vi "Laser.vi"() -> ()   [LabVIEW 2013]
doc: "Пограмма управления мишенью лазерного источника ионов."
uses:
  <vilib>/Utility/error.llb/DialogType.ctl
  <vilib>/Utility/inputDevices.llb/closeJoystick.vi
  <vilib>/Utility/inputDevices.llb/mouseAcquire.vi
panel:
  in  "?":enum32{" Графики", " Настройки соединения"}(tab)
  in  "LiF 3":picture
  in  "LiF 2":picture
  in  "LiF 1":picture
  in  "Дейтерированный полиэтилен":picture
  out "Slide X axis":u8(slide) max=100 scale=0.0..100.0
  out "Slide Y axis":u8(slide) max=50 step=1
  in  "Add Button":bool
  in  "Коорд. Y":u16
  in  "Коорд. X":u16
  in  "Снимок":bool
  in  "Запись в файл":bool
  out "con err":bool caption="Connect"
  out "Con":bool
  out "warning1":string
  out "TCP read data":string
  in  "thickness":u16 step=1
  out "Mouse on Pane pos Horizontal":i32
  out "Mouse on Pane pos Vertical":i32
  out "bytes written":i32
  in  "порт":u16=10001
  in  "IP-адрес":string="159.93.126.157"
  in  "Disconnect":bool caption="Disconn"
  out "Connected":bool
  in  "Connect":bool
  out "TCP error source":string
  in  "stop":bool
  out "read_error_indicator":bool
  in  "Connect 2":bool caption="Connect"
  in  "Компактный вид":bool
  out "resize Fl":bool caption="Disconn"
  in  "flag1":bool caption="Disconn"
  out "x+1":dbl
  out "TCP con ID":refnum<k5>
  # "Дейтерированный полиэтилен"
  # "LiF 1"
  # "LiF 2"
  # "Графит"
types:
  T1 = typedef "DialogType.ctl" = u16
  T2 = typedef "imagedata.ctl" = cluster{"image type":i32, "image depth":i32, "image":u8[], "mask":u8[], "colors":u32[], "Rectangle":cluster{"left":i16, "top":i16, "right":i16, "bottom":i16}}
  T3 = cluster{"Horizontal":i32, "Vertical":i32, "Scrolling":i32}
  T4 = typedef "LVRectTypeDef.ctl" = cluster{"Left":i16, "Top":i16, "Right":i16, "Bottom":i16}
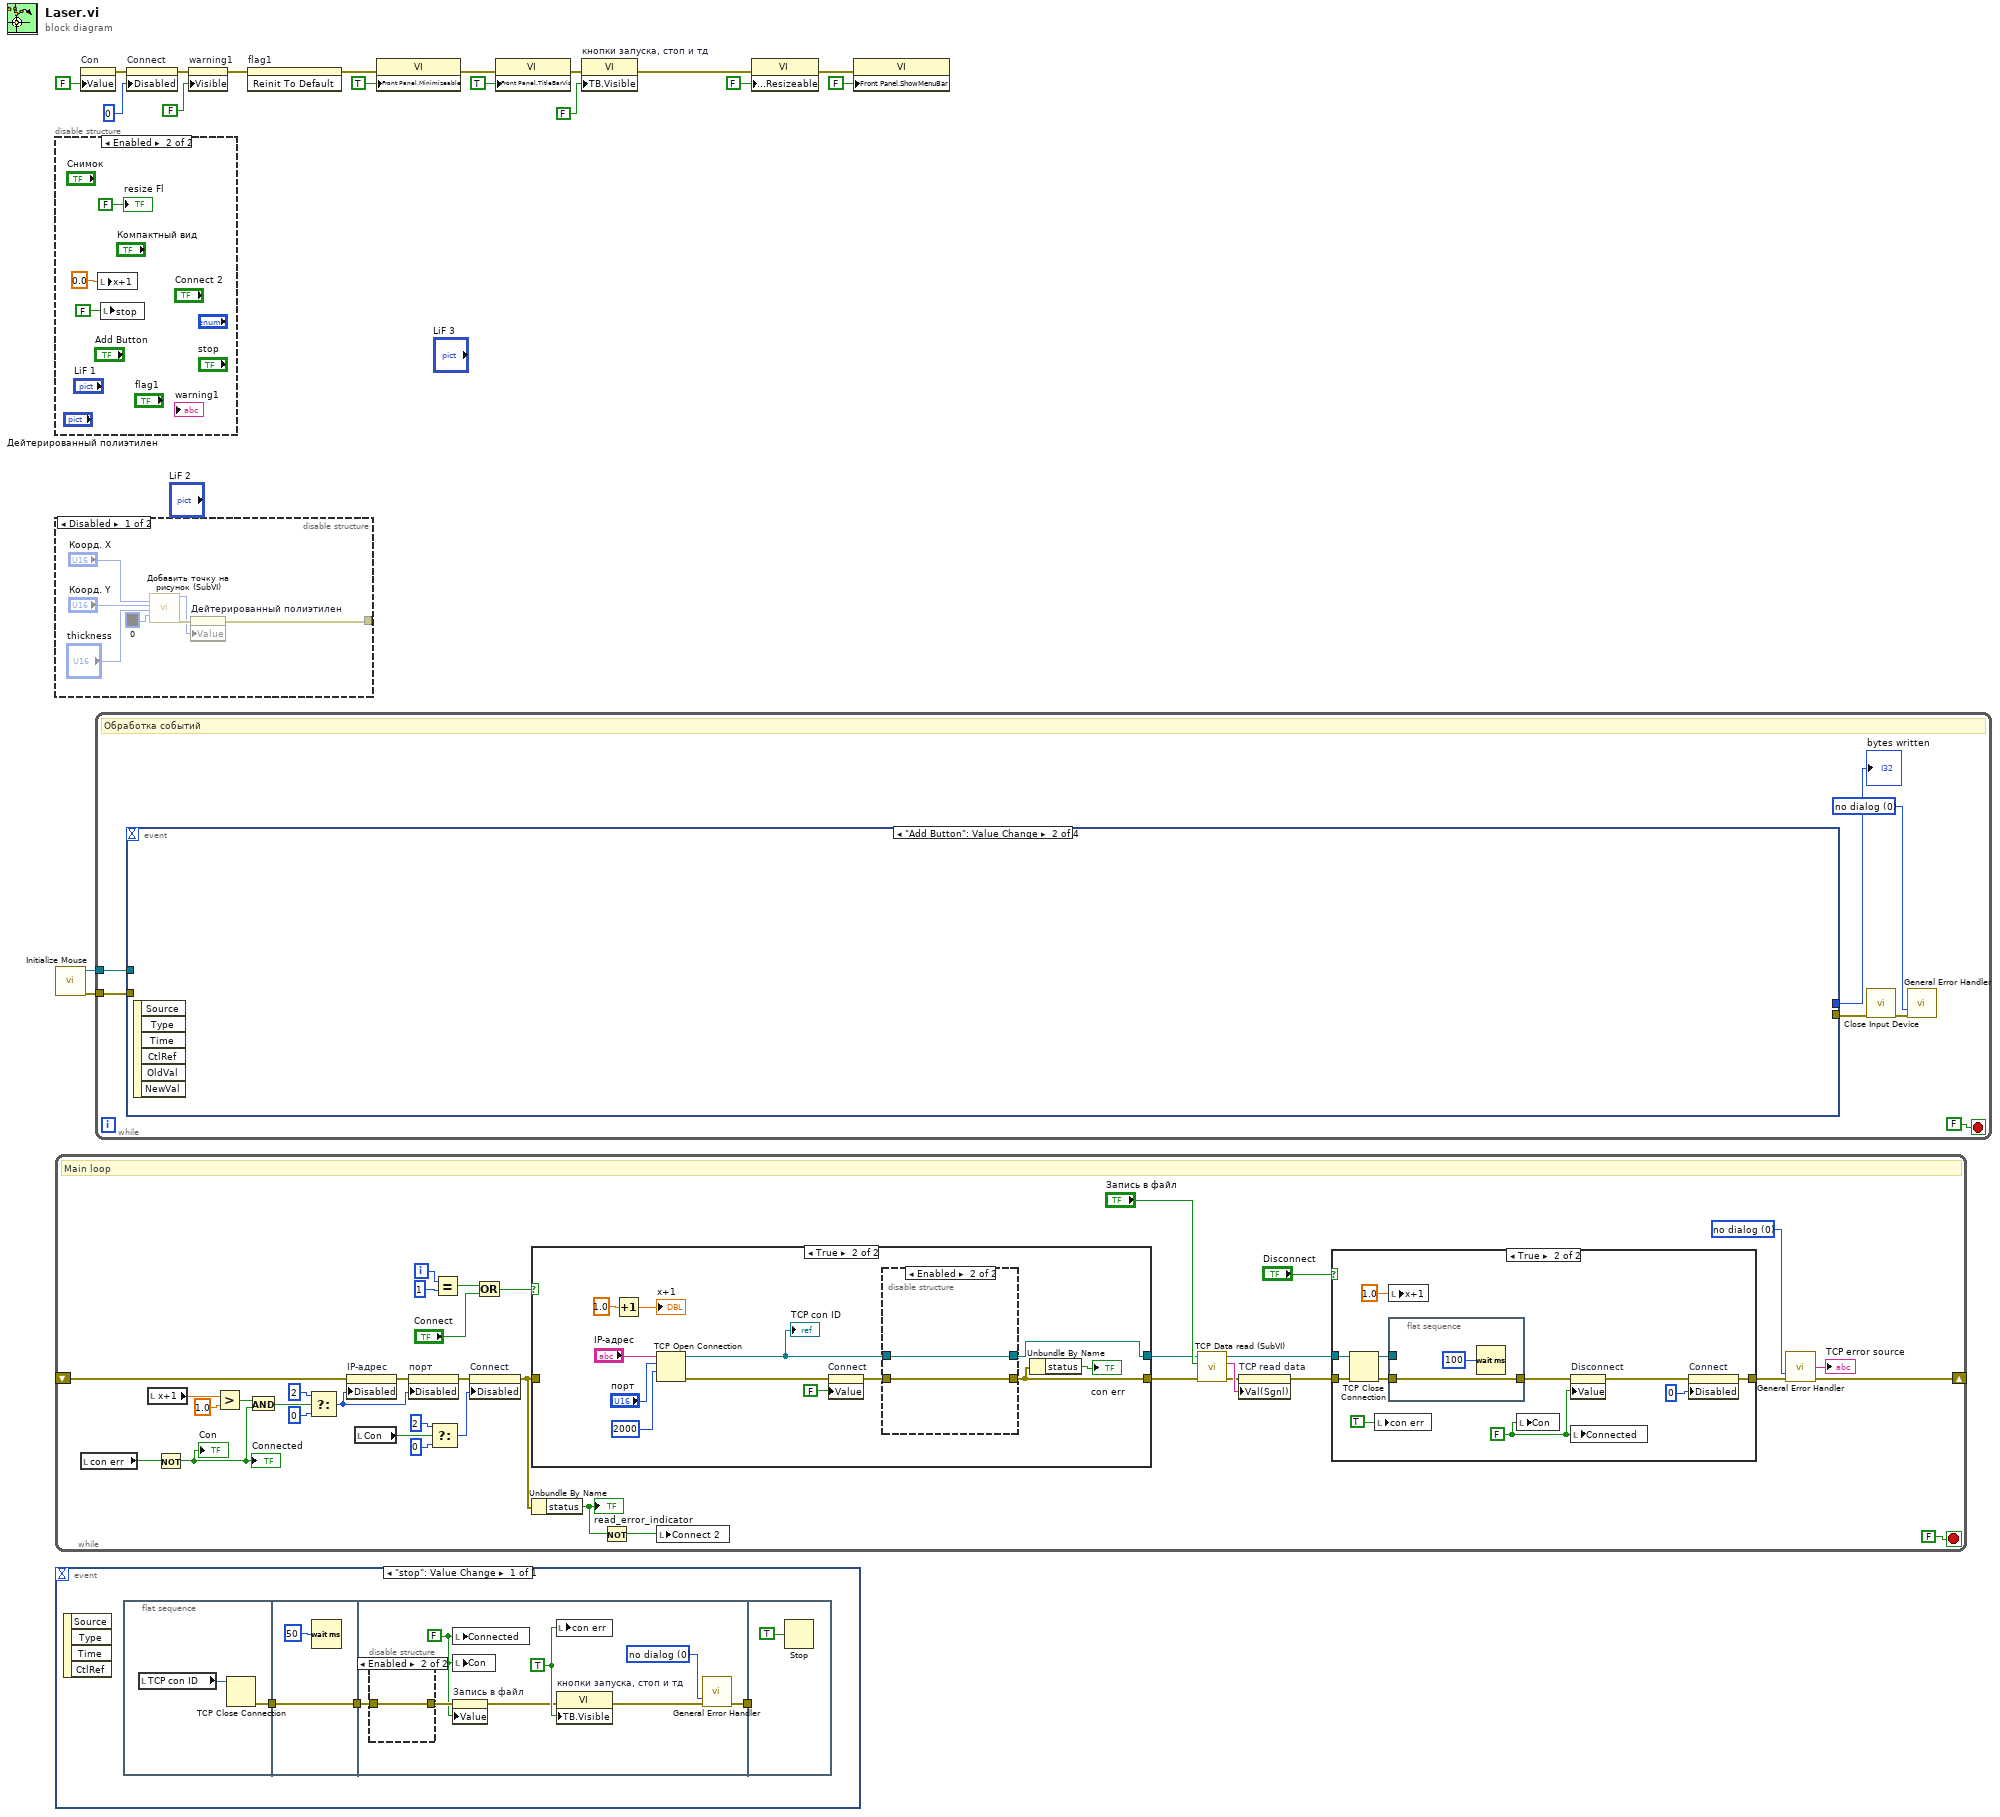
[diagram p0: block diagram]
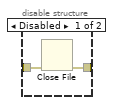
[diagram p4: hidden frame]
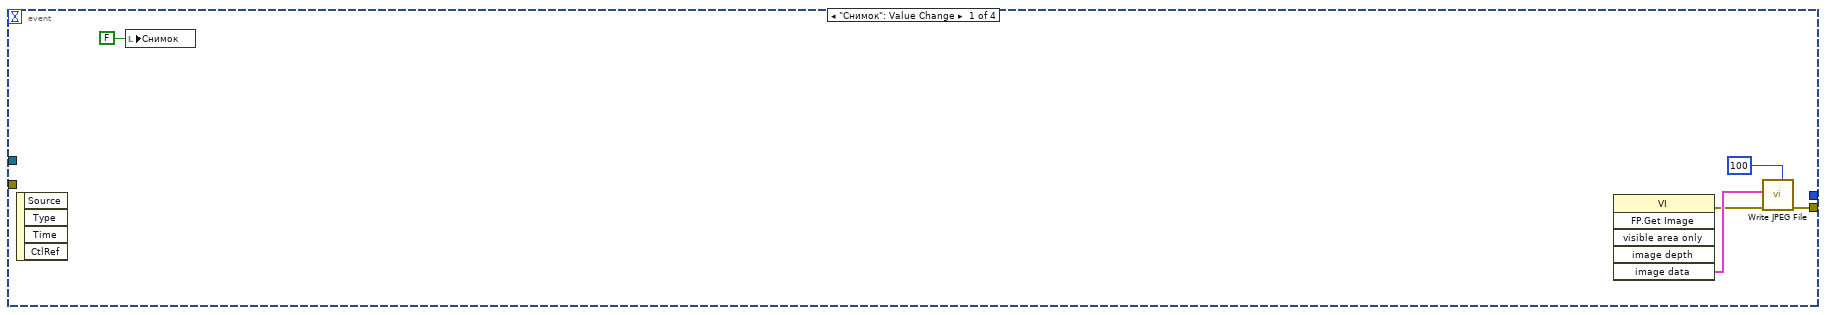
[diagram p5: hidden frame]
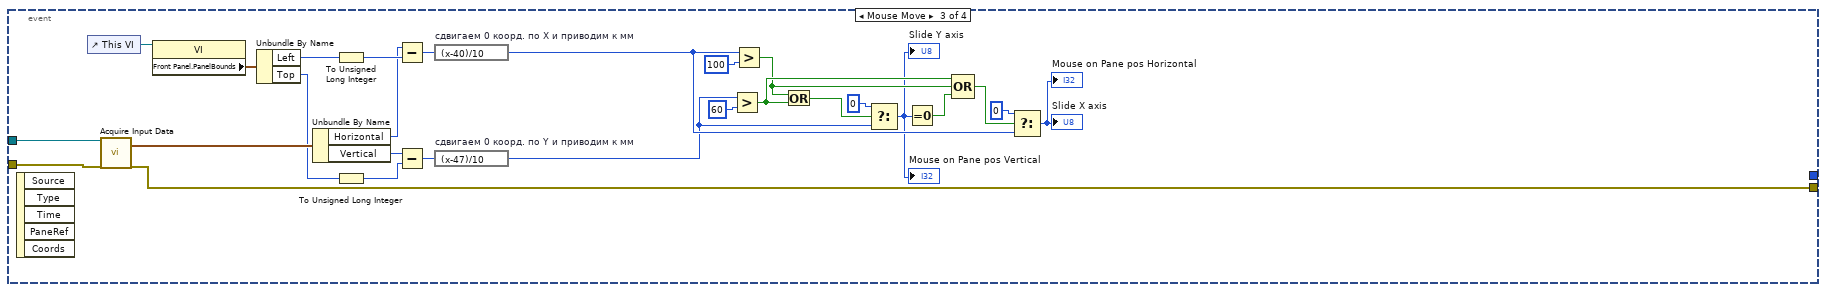
[diagram p6: hidden frame]
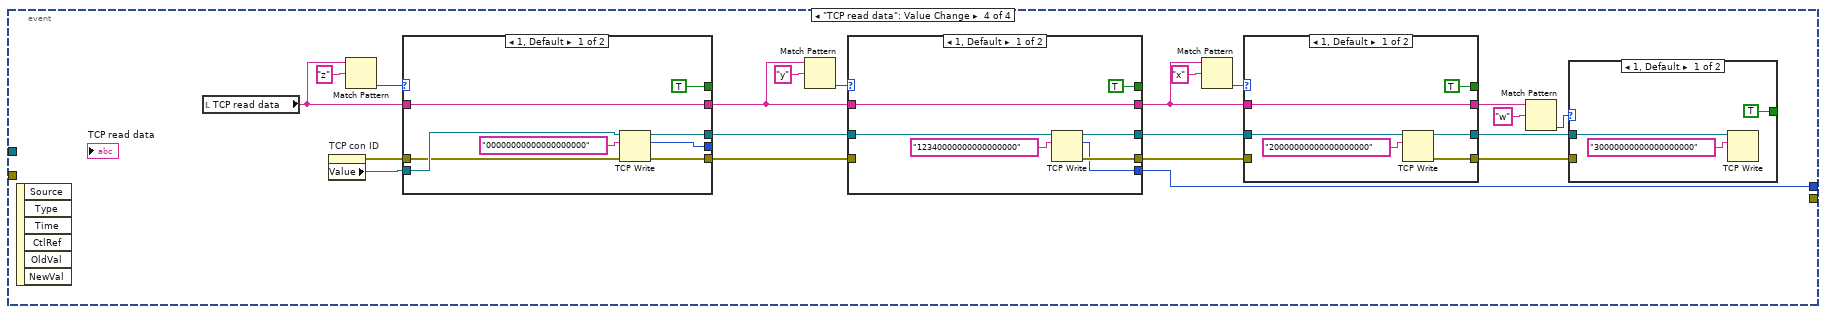
[diagram p7: hidden frame]
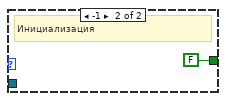
[diagram p8: hidden frame]
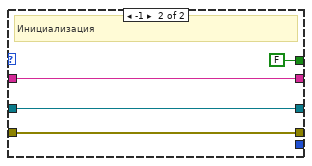
[diagram p9: hidden frame]
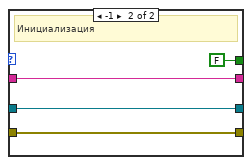
[diagram p10: hidden frame]
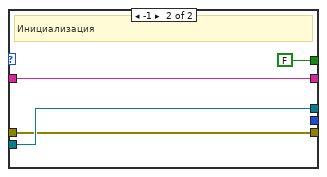
[diagram p11: hidden frame]
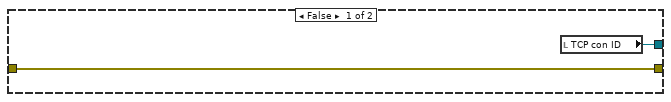
[diagram p12: hidden frame]
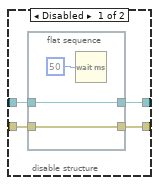
[diagram p13: hidden frame]
diagram:
  n1 = disable-structure shown="Enabled" {
    frame Disabled {
    }
    frame Enabled {
      n2 = local write "x+1"(0.0 ("x+1")) -> ()
      n3 = local write "stop"(FALSE ("Boolean")) -> ()
      "resize Fl" <- FALSE ("resize Fl")
    }
  }
  n4 = disable-structure shown="Disabled" {
    disable-tunnel: [w22 _] -> _
    frame Disabled {
      n5 = call "Добавить точку на рисунок (SubVI).vi"("dot х"="Коорд. X", "dot y"="Коорд. Y", "thickness"="thickness", "цвет"=u32 0) -> ("in picture"=w27:picture, "out picture"=w28:picture, "error out"=w29:errorcluster)  [unwired: 13 in]
      n6 = property on="Дейтерированный полиэтилен" class="Pict"(error in=w29, "Value"=w28) -> (error out=w22:errorcluster)  [unwired: 1 in, 1 out]
    }
    frame Enabled {
    }
  }
  n7 = call <vilib>:"Initialize Mouse.vi"() -> ("error out"=w2:errorcluster, "device ID"=w1:refnum<k1>)  [unwired: 10 in]
  n8 = while {
    shift-right: [w41] -> _
    shift-left: _ -> [w39]
    i -> [w46]
    stop <- FALSE stop-if-true
    w42 = T1 0 items=["no dialog", "OK message", "continue or stop message", "OK message + warnings", "continue/stop + warnings"] ("type of dialog (OK msg:1)")
    # "Main loop"
    n9 = local read "con err"() -> (w63:bool)
    n10 = local read "x+1"() -> (w66:dbl)
    n11 = Not(x=w63) -> (.not. x?=w62:bool)
    "Connected" <- w62
    "Con" <- w62
    n12 = Greater?(x=w66, y=1.0) -> (0:w64:bool)
    n13 = And(x=w64, y=w62) -> (x .and. y?=w53:bool)
    n14 = Select(t=u8 2 ("Disabled"), s=w53, f=u8 0 ("Disabled")) -> (s? t:f=w52:u8)
    n15 = property on="IP-адрес" class="Str"(error in=w39, "Disabled"=w52) -> (error out=w51:errorcluster)  [unwired: 1 in, 1 out]
    n16 = local read "Con"() -> (w59:bool)
    n17 = property on="порт" class="DigNum (strict)"(error in=w51, "Disabled"=w52) -> (error out=w50:errorcluster)  [unwired: 1 in, 1 out]
    n18 = Select(t=u8 2 ("Disabled"), s=w59, f=u8 0 ("Disabled")) -> (s? t:f=w56:u8)
    n19 = Equal?(x=w46, y=1) -> (x = y?=w47:bool)
    n20 = property on="Connect" class="Bool (strict)"(error in=w50, "Disabled"=w56) -> (error out=w44:errorcluster)  [unwired: 1 in, 1 out]
    n21 = Or(x=w47, y="Connect") -> (x .or. y?=w49:bool)
    n22 = case shown="True" w49 {
      tunnel: [w68 w69] -> w37
      tunnel: [w67 w71] -> w35
      tunnel: w44 -> [w68 _]
      frame False {
        n23 = local read "TCP con ID"() -> (w67:refnum<k5>)
      }
      frame True {
        n24 = Increment(x=1.0) -> (x+1=→"x+1":dbl)
        n25 = TCP Open Connection(address="IP-адрес", remote port or service name="порт", timeout ms (60000)=2000) -> (connection ID=w72:refnum<k5>, error out=w74:errorcluster)  [unwired: 1 in, 1 out]
        "TCP con ID" <- w72
        n26 = property on="Connect" class="Bool (strict)"(error in=w74, "Value"=FALSE ("Connect")) -> (error out=w73:errorcluster)  [unwired: 1 in, 1 out]
        n27 = disable-structure shown="Enabled" {
          disable-tunnel: w73 -> [w84 w88]
          disable-tunnel: w72 -> [w83 w89]
          disable-tunnel: [w82 w89] -> w71
          disable-tunnel: [w81 w88] -> w69
          frame Disabled {
            n28 = flat-sequence {
              tunnel: w84 -> [w86]
              tunnel: [w86] -> w81
              tunnel: w83 -> [w85]
              tunnel: [w85] -> w82
              frame #0 {
                n29 = Wait (ms)(milliseconds to wait=u32 50) -> ()  [unwired: 1 out]
              }
            }
          }
          frame Enabled {
          }
        }
        n30 = Unbundle By Name(w69) -> ("status"=→"con err":bool)
      }
    }
    n31 = Unbundle By Name(w44) -> ("status"=w38:bool)
    "read_error_indicator" <- w38
    n32 = Not(x=w38) -> (.not. x?=w61:bool)
    n33 = local write "Connect 2"(w61) -> ()
    n34 = call "TCP Data read (SubVI).vi"("error in (no error)"=w37, "Запись в файл"="Запись в файл", "TCP Network Connection in"=w35) -> ("error out"=w31:errorcluster, "Read data"=w32:string, "TCP Network Connection out"=w34:refnum<k5>)  [unwired: 5 in, 1 out]
    n35 = property on="TCP read data" class="Str"(error in=w31, "Val(Sgnl)"=w32) -> (error out=w30:errorcluster)  [unwired: 1 in, 1 out]
    n36 = case shown="True" "Disconnect" {
      tunnel: [_ w92] -> w40
      tunnel: w30 -> [_ w91]
      tunnel: w34 -> [_ w90]
      frame False {
      }
      frame True {
        w93 = FALSE ("Disconnect")
        n37 = TCP Close Connection(connection ID=w90, error in (no error)=w91) -> (connection ID out=w96:refnum<k5>, error out=w95:errorcluster)  [unwired: 1 out]
        n38 = local write "con err"(TRUE ("con err")) -> ()
        n39 = local write "x+1"(1.0 ("1")) -> ()
        n40 = flat-sequence {
          tunnel: w96 -> [_]
          tunnel: w95 -> [w101]
          tunnel: [w101] -> w94
          frame #0 {
            n41 = Wait (ms)(milliseconds to wait=u32 100) -> ()  [unwired: 1 out]
          }
        }
        n42 = local write "Con"(w93) -> ()
        n43 = property on="Disconnect" class="Bool (strict)"(error in=w94, "Value"=w93) -> (error out=w97:errorcluster)  [unwired: 1 in, 1 out]
        n44 = local write "Connected"(w93) -> ()
        n45 = property on="Connect" class="Bool (strict)"(error in=w97, "Disabled"=u8 0) -> (error out=w92:errorcluster)  [unwired: 1 in, 1 out]
      }
    }
    n46 = call <vilib>:"General Error Handler.vi"("type of dialog (OK msg:1)"=w42, "error in (no error)"=w40) -> ("source out"=→"TCP error source":string, "error out"=w41:errorcluster)  [unwired: 12 out]
  }
  n47 = event shown="[0] \"stop\": Value Change" {
    selector: _ -> [_]
    dyn-events: _ -> [_]
    timeout: _ -> [_]
    event "stop": Value Change {
      n48 = event-data() -> ()  [unwired: 5 out]
      n49 = flat-sequence {
        tunnel: [w106] -> w105
        tunnel: w105 -> [w109]
        tunnel: [w109] -> w104
        tunnel: w104 -> [w112]
        tunnel: [w110] -> w103
        tunnel: w103 -> [_]
        frame #0 {
          n50 = local read "TCP con ID"() -> (w107:refnum<k5>)
          n51 = TCP Close Connection(connection ID=w107) -> (error out=w106:errorcluster)  [unwired: 1 in, 2 out]
        }
        frame #1 {
          n52 = Wait (ms)(milliseconds to wait=u32 50) -> ()  [unwired: 1 out]
        }
        frame #2 {
          w113 = T1 0 items=["no dialog", "OK message", "continue or stop message", "OK message + warnings", "continue/stop + warnings"] ("type of dialog (OK msg:1)")
          w116 = FALSE ("Запись в файл")
          w115 = TRUE ("Tool Bar:Visible")
          n53 = disable-structure shown="Enabled" {
            disable-tunnel: [w119 w120] -> w117
            disable-tunnel: w112 -> [w118 w120]
            frame Disabled {
              n54 = Close File(error in=w118) -> (error out=w119:errorcluster)  [unwired: 1 in, 1 out]
            }
            frame Enabled {
            }
          }
          n55 = local write "Connected"(w116) -> ()
          n56 = local write "Con"(w116) -> ()
          n57 = property on="Запись в файл" class="Bool (strict)"(error in=w117, "Value"=w116) -> (error out=w114:errorcluster)  [unwired: 1 in, 1 out]
          n58 = local write "con err"(w115) -> ()
          n59 = property on="кнопки запуска, стоп и тд" class="VI"(error in=w114, "TB.Visible"=w115) -> (error out=w111:errorcluster)  [unwired: 1 in, 1 out]
          n60 = call <vilib>:"General Error Handler.vi"("type of dialog (OK msg:1)"=w113, "error in (no error)"=w111) -> ("error out"=w110:errorcluster)  [unwired: 13 out]
        }
        frame #3 {
          n61 = Stop(stop? (T)=TRUE) -> ()
        }
      }
    }
  }
  n62 = property on="Con" class="Bool (strict)"("Value"=FALSE ("Connected")) -> (error out=w5:errorcluster)  [unwired: 2 in, 1 out]
  n63 = while {
    tunnel: w2 -> [w126]
    tunnel: w1 -> [w125]
    stop <- FALSE stop-if-true
    w127 = T1 0 items=["no dialog", "OK message", "continue or stop message", "OK message + warnings", "continue/stop + warnings"] ("type of dialog (OK msg:1)")
    # "Обработка событий"
    n64 = event shown="[1] \"Add Button\": Value Change" {
      selector: _ -> [_ _ _ _]
      dyn-events: _ -> [_ _ _ _]
      timeout: _ -> [_ _ _ _]
      tunnel: [w129 _ w153 _] -> w124
      tunnel: w126 -> [_ _ w159 _]
      tunnel: w125 -> [_ _ w160 _]
      tunnel: [_ _ _ w161] -> w122
      event "Снимок": Value Change {
        n65 = event-data() -> ()  [unwired: 5 out]
        n66 = local write "Снимок"(FALSE ("Снимок")) -> ()
        n67 = invoke class="VI" method="FP.Get Image"() -> (error out=w130:errorcluster, "image data"=w131:T2)  [unwired: 6 in, 4 out]
        n68 = call <vilib>:"Write JPEG File.vi"("quality (80)"=100, "error in (no error)"=w130, "image data"=w131) -> ("error out"=w129:errorcluster)  [unwired: 1 in, 7 out]
      }
      event "Add Button": Value Change {
        n69 = event-data() -> ()  [unwired: 7 out]
      }
      event Mouse Move {
        n70 = event-data() -> ()  [unwired: 6 out]
        n71 = control-ref of="This VI"() -> (w157:refnum<vi>)
        n72 = call-poly <vilib>:"Acquire Input Data.vi"("device ID"=w160, "error in (no error)"=w159) -> ("axis info"=w158:T3, "error out"=w153:errorcluster)  [unwired: 14 in, 2 out]
        n73 = property class="VI"(reference=w157) -> ("Front Panel.PanelBounds"=w156:T4)  [unwired: 1 in, 2 out]
        n74 = Unbundle By Name(w156) -> ("Left"=w155:i16, "Top"=w154:i16)
        n75 = Unbundle By Name(w158) -> ("Horizontal"=w151:i32, "Vertical"=w149:i32)
        n76 = To Unsigned Long Integer(number=w155) -> (unsigned 32bit integer=w152:u32)
        n77 = To Unsigned Long Integer(number=w154) -> (unsigned 32bit integer=w150:u32)
        n78 = Subtract(x=w151, y=w152) -> (x-y=w148:u32)
        n79 = Subtract(x=w149, y=w150) -> (x-y=w147:u32)
        n80 = expression code="(x-40)/10" "сдвигаем 0 коорд. по X и приводим к мм"(w148) -> (w142:u32)
        n81 = expression code="(x-47)/10" "сдвигаем 0 коорд. по Y и приводим к мм"(w147) -> (w141:u32)
        n82 = Greater?(x=w141, y=60) -> (0:w139:bool)
        n83 = Greater?(x=w142, y=100) -> (0:w138:bool)
        n84 = Or(x=w138, y=w139) -> (x .or. y?=w140:bool)
        n85 = Select(t=0, s=w140, f=w141) -> (s? t:f=w135:u32)
        "Mouse on Pane pos Vertical" <- w135
        "Slide Y axis" <- w135
        n86 = Equal To 0?(x=w135) -> (x = 0?=w137:bool)
        n87 = Compound Arithmetic op=OR(w139, w138, w137) -> (w136:bool)
        n88 = Select(t=0, s=w136, f=w142) -> (s? t:f=→"Mouse on Pane pos Horizontal" →"Slide X axis":u32)
      }
      event "TCP read data": Value Change {
        n89 = event-data() -> ()  [unwired: 7 out]
        n90 = local read "TCP read data"() -> (w178:string)
        n91 = property on="TCP con ID" class="Ref (strict)"() -> (error out=w177:errorcluster, "Value"=w162:refnum<k5>)  [unwired: 2 in, 1 out]
        n92 = Match Pattern(string=w178, regular expression="z") -> (offset past match=w163:i32)  [unwired: 1 in, 3 out]
        n93 = case shown="1, Default" w163 {
          tunnel: w162 -> [w212 w217]
          tunnel: [TRUE ("Boolean") FALSE ("Boolean")] -> _
          tunnel: [w210 w216] -> w173
          tunnel: [w211 w217] -> w171
          tunnel: w177 -> [w209 w216]
          tunnel: [w208 w215] -> w179
          tunnel: w178 -> [w208 w215]
          tunnel: [w207 _] -> _
          frame 1, Default {
            n94 = TCP Write(connection ID=w212, data in="00000000000000000000", error in (no error)=w209) -> (connection ID out=w211:refnum<k5>, bytes written=w207:i32, error out=w210:errorcluster)  [unwired: 1 in]
          }
          frame -1 {
            # "Инициализация"
          }
        }
        n95 = Match Pattern(string=w179, regular expression="y") -> (offset past match=w170:i32)  [unwired: 1 in, 3 out]
        n96 = case shown="1, Default" w170 {
          tunnel: [w190 w194] -> w174
          tunnel: [TRUE ("Boolean") FALSE ("Boolean")] -> _
          tunnel: w171 -> [w189 w195]
          tunnel: w173 -> [_ w194]
          tunnel: [w188 w195] -> w176
          tunnel: [w187 w193] -> w181
          tunnel: w179 -> [w187 w193]
          tunnel: [w186 _] -> w161
          frame 1, Default {
            n97 = TCP Write(connection ID=w189, data in="12340000000000000000") -> (connection ID out=w188:refnum<k5>, bytes written=w186:i32, error out=w190:errorcluster)  [unwired: 2 in]
          }
          frame -1 {
            # "Инициализация"
          }
        }
        n98 = Match Pattern(string=w181, regular expression="x") -> (offset past match=w166:i32)  [unwired: 1 in, 3 out]
        n99 = case shown="1, Default" w166 {
          tunnel: [w200 w204] -> w175
          tunnel: [TRUE ("Boolean") FALSE ("Boolean")] -> _
          tunnel: [w198 w205] -> w172
          tunnel: w174 -> [_ w204]
          tunnel: w176 -> [w199 w205]
          tunnel: [w197 w203] -> w180
          tunnel: w181 -> [w197 w203]
          frame 1, Default {
            n100 = TCP Write(connection ID=w199, data in="20000000000000000000") -> (connection ID out=w198:refnum<k5>, error out=w200:errorcluster)  [unwired: 2 in, 1 out]
          }
          frame -1 {
            # "Инициализация"
          }
        }
        n101 = Match Pattern(string=w180, regular expression="w") -> (offset past match=w167:i32)  [unwired: 1 in, 3 out]
        n102 = case shown="1, Default" w167 {
          tunnel: [TRUE ("Boolean") FALSE ("Boolean")] -> _
          tunnel: w172 -> [w182 _]
          tunnel: w175 -> [_ _]
          frame 1, Default {
            n103 = TCP Write(connection ID=w182, data in="30000000000000000000") -> ()  [unwired: 2 in, 3 out]
          }
          frame -1 {
            # "Инициализация"
          }
        }
      }
    }
    "bytes written" <- w122
    n104 = call-poly <vilib>:"Close Input Device.vi"("error in (no error)"=w124) -> ("error out"=w123:errorcluster)  [unwired: 9 in]
    n105 = call <vilib>:"General Error Handler.vi"("type of dialog (OK msg:1)"=w127, "error in (no error)"=w123) -> ()  [unwired: 9 in, 5 out]
  }
  n106 = property on="Connect" class="Bool (strict)"(error in=w5, "Disabled"=u8 0) -> (error out=w10:errorcluster)  [unwired: 1 in, 1 out]
  n107 = property on="warning1" class="Str"(error in=w10, "Visible"=FALSE) -> (error out=w3:errorcluster)  [unwired: 1 in, 1 out]
  n108 = invoke on="flag1" class="Bool (strict)" method="Reinit To Default"(error in=w3) -> (error out=w4:errorcluster)  [unwired: 2 in, 2 out]
  n109 = property class="VI"(error in=w4, "Front Panel.Minimizeable"=TRUE ("Front Panel Window:Minimizable")) -> (error out=w9:errorcluster)  [unwired: 1 in, 1 out]
  n110 = property class="VI"(error in=w9, "Front Panel.TitleBarVis"=TRUE ("Front Panel Window:Title Bar Visible")) -> (error out=w8:errorcluster)  [unwired: 1 in, 1 out]
  n111 = property on="кнопки запуска, стоп и тд" class="VI"(error in=w8, "TB.Visible"=FALSE ("Tool Bar:Visible")) -> (error out=w7:errorcluster)  [unwired: 1 in, 1 out]
  n112 = property class="VI"(error in=w7, "Front Panel.Resizeable"=FALSE ("Front Panel Window:Resizable")) -> (error out=w6:errorcluster)  [unwired: 1 in, 1 out]
  n113 = property class="VI"(error in=w6, "Front Panel.ShowMenuBar"=FALSE ("Front Panel Window:Show Menu Bar")) -> ()  [unwired: 1 in, 2 out]
